vi "DiffDrivePoseEst_VisionCorrect_Callback.vi"(8 "ExtraPassedData":variant, 9 "Y":T2, 10 "U":T2, 11 "in UNSCENTED_KALMAN_FILTER":T1) -> (0 "Error":bool, 3 "out UNSCENTED_KALMAN_FILTER":T1)   [LabVIEW 2019, in "Trajectory_Library.lvlib"]
doc: "This set of functions is deprecated. Suggest using the new Diff Drive Pose Est 2 instead.\n\nFunction used by LatencyCompensator_ApplyPastGlobalMeasurement\n\nThis is a work in progress!!"
uses:
  Trajectory_Library.lvlib
  <vilib>/Analysis/Matrix/Datatypes/RealMatrix.ctl
  TypeDef/UNSCENTED_KALMAN_FILTER.ctl
  TypeDef/MERWE_SCALED_SIGMA_PTS.ctl
  TypeDef/CALLBACK_FUNC_TYPE.ctl
  <vilib>/Analysis/Matrix/NI_Matrix.lvlib
panel:
  in  "Cluster":cluster{"VisionDiscreteR":T2}
  # "State Estimate <Statess,1>"
  # "<States, States>"
  # "<States, ?>"
  # "<Statess,  States>"
  # "<Outputs, Outputs>"
  # "<?, 1>"
  # "<?, 1>"
  # "State Estimate <Statess,1>"
  # "<States, States>"
  # "<States, ?>"
  # "<Statess,  States>"
  # "<Outputs, Outputs>"
  # "<?, 1>"
  # "<?, 1>"
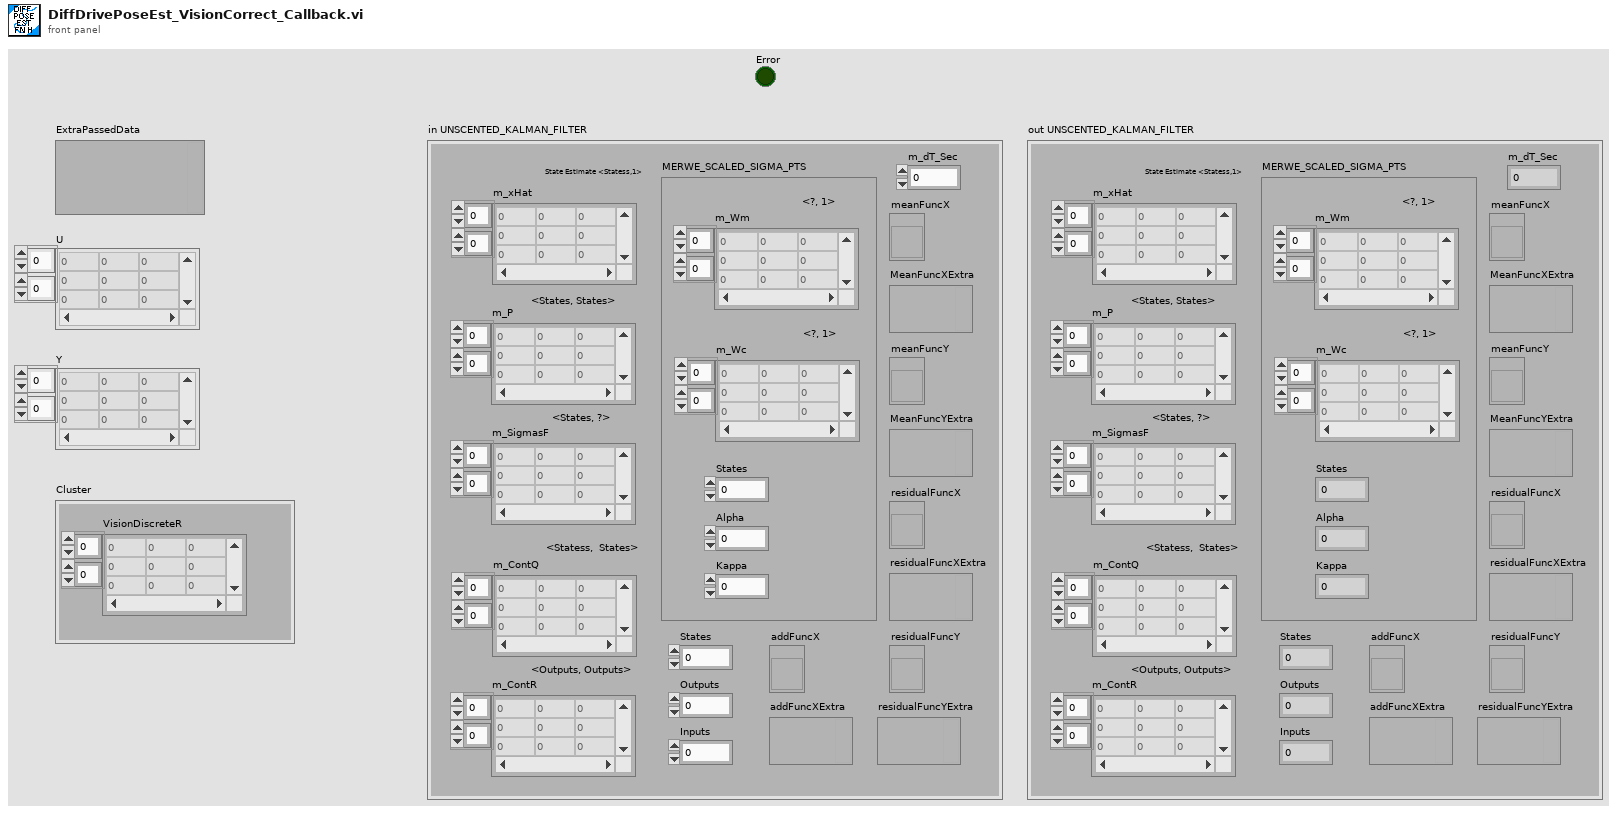
[diagram p1: front panel]
types:
  T1 = typedef "Trajectory_Library.lvlib/UNSCENTED_KALMAN_FILTER.ctl" = cluster{"m_P":T2, "m_xHat":T2, "States":i32, "Outputs":i32, "m_ContR":T2, "m_ContQ":T2, "m_SigmasF":T2, "m_dT_Sec":dbl, "MERWE_SCALED_SIGMA_PTS":T3, "meanFuncX":T4, "meanFuncY":T4, "residualFuncX":T4, "residualFuncY":T4, "addFuncX":T4, "addFuncXExtra":variant, "residualFuncYExtra":variant, "residualFuncXExtra":variant, "MeanFuncYExtra":variant, "MeanFuncXExtra":variant, "Inputs":i32}
  T2 = typedef "NI_Matrix.lvlib/RealMatrix.ctl" = dbl[][]
  T3 = typedef "Trajectory_Library.lvlib/MERWE_SCALED_SIGMA_PTS.ctl" = cluster{"m_Wm":T2, "States":i32, "Alpha":dbl, "m_Wc":T2, "Kappa":i32}
  T4 = typedef "Trajectory_Library.lvlib/CALLBACK_FUNC_TYPE.ctl" = refnum<vi>
  T5 = typedef "Trajectory_Library.lvlib/UNSCENTED_KALMAN_CORRECT_FUNC_GROUP.ctl" = cluster{"H_Func":T4, "meanFuncY":T4, "residualFuncY":T4, "residualFuncX":T4, "addFuncX":T4, "H_FuncExtra":variant, "MeanFuncYExtra":variant, "residualFuncYExtra":variant, "residualFuncXExtra":variant, "addFuncXExtra":variant}
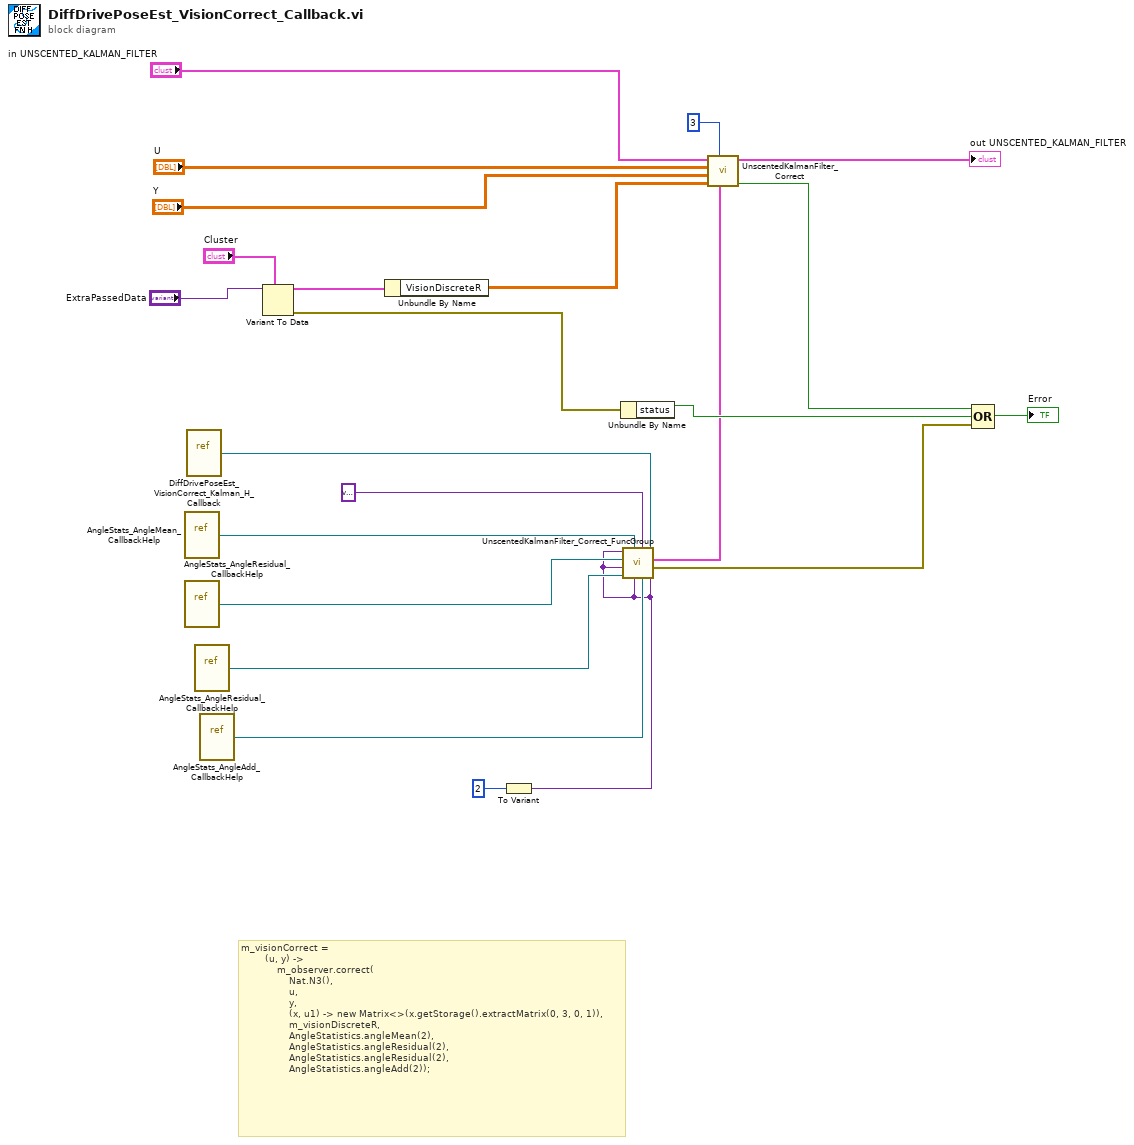
[diagram p0: block diagram]
diagram:
  # "m_visionCorrect =\n        (u, y) ->\n            m_observer.correct(\n                Nat.N3(),\n                u,\n                y,\n                (x, u1) -> new Matrix<>(x.getStorage().extractMatrix(0, 3, 0, 1)),\n                m_visionDiscreteR,\n                AngleStatistics.angleMean(2),\n                AngleStatistics.angleResidual(2),\n                AngleStatistics.angleResidual(2),\n                AngleStatistics.angleAdd(2));"
  n1 = vi-ref "AngleStats_AngleMean_CallbackHelp.vi"() -> (w7:refnum<vi>)
  n2 = vi-ref "AngleStats_AngleResidual_CallbackHelp.vi"() -> (w8:refnum<vi>)
  n3 = vi-ref "DiffDrivePoseEst_VisionCorrect_Kalman_H_Callback.vi"() -> (w1:refnum<vi>)
  n4 = vi-ref "AngleStats_AngleResidual_CallbackHelp.vi"() -> (w9:refnum<vi>)
  n5 = vi-ref "AngleStats_AngleAdd_CallbackHelp.vi"() -> (w10:refnum<vi>)
  n6 = Variant To Data(type="Cluster", Variant="ExtraPassedData") -> (data=w21:cluster{"VisionDiscreteR":T2}, error out=w18:errorcluster)  [unwired: 1 in]
  n7 = Unbundle By Name(w21) -> ("VisionDiscreteR"=w12:T2)
  n8 = To Variant(anything=2) -> (Variant=w4:variant)
  n9 = Unbundle By Name(w18) -> ("status"=w17:bool)
  n10 = call "UnscentedKalmanFilter_Correct_FuncGroup.vi"("addFuncXExtra"=w4, "H_Func"=w1, "AddFuncX"=w10, "H_FuncExtra"=variant ("F_Func_ExtraData"), "residualFuncXExtra"=w4, "MeanFuncY"=w7, "ResidualFuncX"=w9, "residualFuncYExtra"=w4, "ResidualFuncY"=w8, "MeanFuncYExtra"=w4) -> ("Error"=w6:errorcluster, "UNSCENTED_KALMAN_CORRECT_FUNC_GROUP"=w13:T5)
  n11 = call "UnscentedKalmanFilter_Correct.vi"("UNSCENTED_KALMAN_CORRECT_FUNC_GROUP"=w13, "Rows"=3, "R"=w12, "Y"="Y", "U"="U", "in UnscentedKalmanFiilter"="in UNSCENTED_KALMAN_FILTER") -> ("Error"=w16:bool, "out UnscentedKalmanFiilter"=→"out UNSCENTED_KALMAN_FILTER":T1)  [unwired: 4 in]
  n12 = Compound Arithmetic op=OR(w16, w17, w6) -> (→"Error":bool)
